vi "DHT22_and_photo.vi"() -> ()   [LabVIEW 2013]
uses:
  <vilib>/Instr/_visa.llb/VISA Configure Serial Port (Instr).vi
panel:
  out "Light Sensor":dbl[](graph)
  out "Light Intensity (a.u.)":dbl
  out "Waveform Chart 2":dbl[](graph)
  out "Temp (C)":dbl
  out "Waveform Chart":dbl[](graph)
  out "Humidity (%)":dbl
  in  "stop":bool
  # "Arduino Temp, Humidity, and Light Sensing"
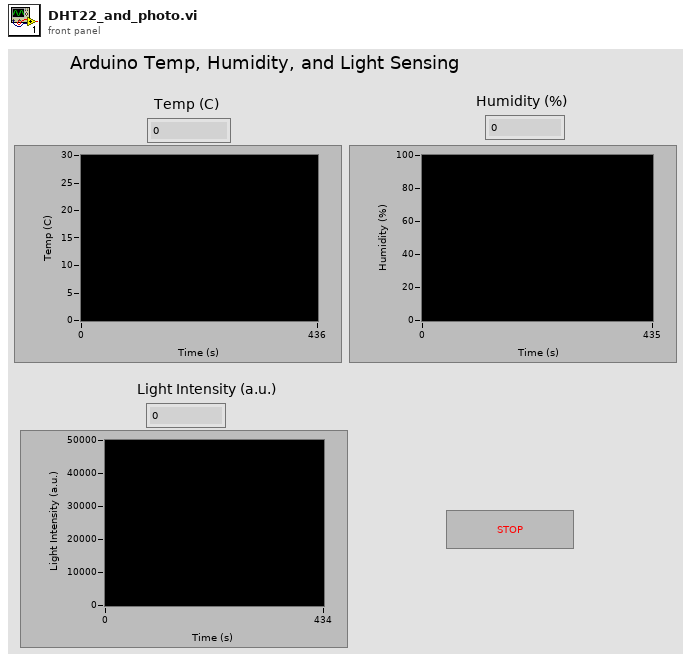
[diagram p1: front panel]
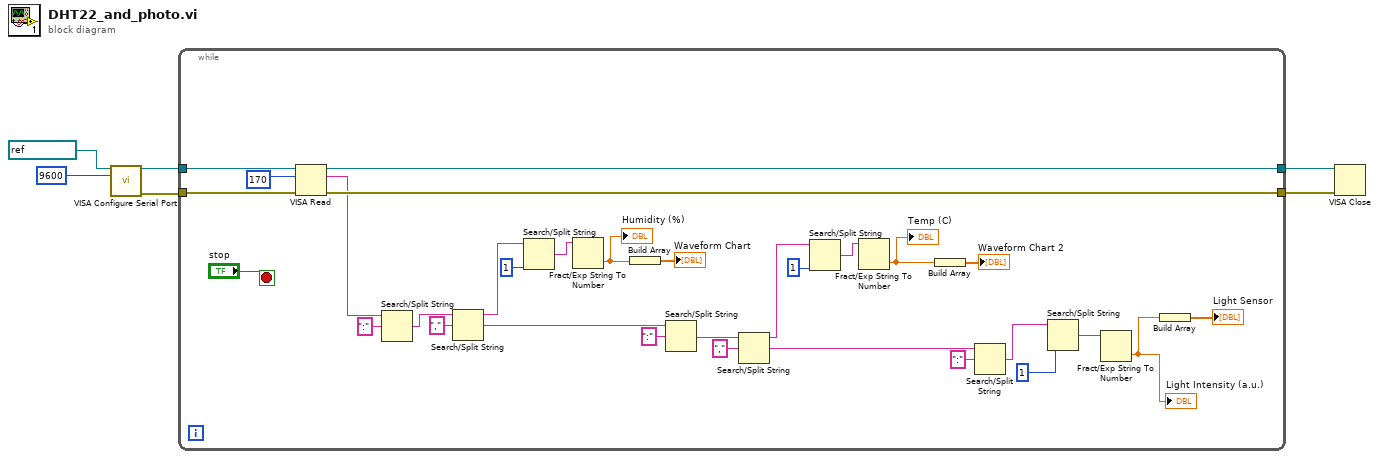
[diagram p0: block diagram]
diagram:
  n1 = call-poly "VISA Configure Serial Port"("VISA resource name"=refnum<visa-resource-name> "COM12", "baud rate (9600)"=u32 9600) -> ("VISA resource name out"=w3:refnum<visa-resource-name>, "error out"=w4:errorcluster)  [unwired: 12 in]
  n2 = while {
    tunnel: w3 -> [w33]
    tunnel: w4 -> [w32]
    tunnel: [w36] -> w6
    tunnel: [w35] -> w5
    stop <- "stop" stop-if-true
    n3 = VISA Read(VISA resource name=w33, byte count=u32 170, error in (no error)=w32) -> (VISA resource name out=w36:refnum<visa-resource-name>, read buffer=w31:string, error out=w35:errorcluster)  [unwired: 1 out]
    n4 = Search/Split String(string=w31, search string/char (-)=":") -> (match + rest of string=w28:string)  [unwired: 1 in, 2 out]
    n5 = Search/Split String(string=w28, search string/char (-)=",") -> (substring before match=w23:string, match + rest of string=w27:string)  [unwired: 1 in, 1 out]
    n6 = Search/Split String(string=w23, offset (0)=1) -> (match + rest of string=w21:string)  [unwired: 1 in, 2 out]
    n7 = Fract/Exp String To Number(string=w21) -> (number=w20:dbl)  [unwired: 3 in, 1 out]
    "Humidity (%)" <- w20
    n8 = Build Array(w20) -> (→"Waveform Chart":dbl[])
    n9 = Search/Split String(string=w27, search string/char (-)=":") -> (match + rest of string=w24:string)  [unwired: 1 in, 2 out]
    n10 = Search/Split String(string=w24, search string/char (-)=",") -> (substring before match=w15:string, match + rest of string=w11:string)  [unwired: 1 in, 1 out]
    n11 = Search/Split String(string=w15, offset (0)=1) -> (match + rest of string=w17:string)  [unwired: 1 in, 2 out]
    n12 = Fract/Exp String To Number(string=w17) -> (number=w18:dbl)  [unwired: 3 in, 1 out]
    "Temp (C)" <- w18
    n13 = Build Array(w18) -> (→"Waveform Chart 2":dbl[])
    n14 = Search/Split String(string=w11, search string/char (-)=":") -> (match + rest of string=w9:string)  [unwired: 1 in, 2 out]
    n15 = Search/Split String(string=w9, offset (0)=1) -> (match + rest of string=w8:string)  [unwired: 1 in, 2 out]
    n16 = Fract/Exp String To Number(string=w8) -> (number=w7:dbl)  [unwired: 3 in, 1 out]
    "Light Intensity (a.u.)" <- w7
    n17 = Build Array(w7) -> (→"Light Sensor":dbl[])
  }
  n18 = VISA Close(VISA resource name=w6, error in (no error)=w5) -> ()  [unwired: 1 out]
